vi "Rohwerte skalieren Kalibrieren.vi"(6 "CAL-Daten":T1={"O2 Null"=0.0, "O2 Steil"=[1.0, 1.0, 1.0, 1.0]}, 11 "GasValue":sgl[](array[numeric])) -> (3 "Kalibrierte Rohwerte":sgl[](array[numeric]))   [LabVIEW 2020, in "ABB-EL3000.lvlib" / "PMA.lvlib" / "Kalibrieren.lvlib"]
uses:
  Kalibrieren.lvlib
  Allgemeine VI/CAL-Daten PMA.ctl
  Allgemeine VI/Allgemeine VI.lvlib
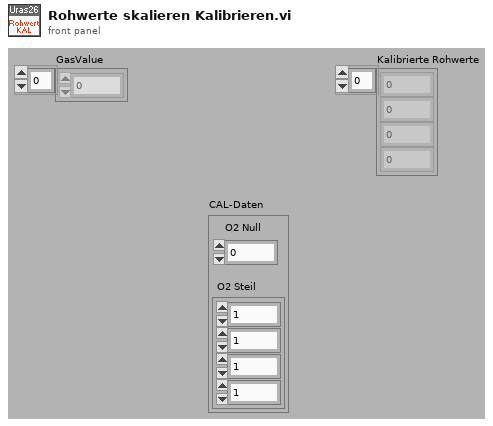
[diagram p1: front panel]
types:
  T1 = typedef "ABB-EL3000.lvlib/Allgemeine VI.lvlib/CAL-Daten PMA.ctl" = cluster{"O2 Null":sgl, "O2 Steil":sgl[]}
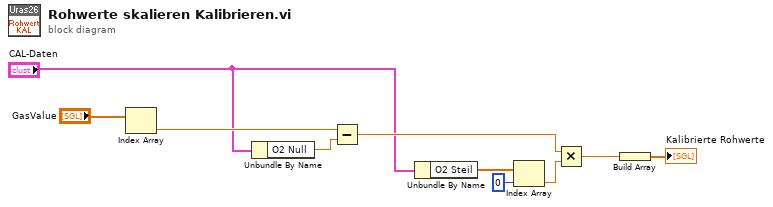
[diagram p0: block diagram]
diagram:
  n1 = Index Array(array="GasValue") -> (element=w3:sgl)  [unwired: 1 in]
  n2 = Unbundle By Name("CAL-Daten") -> ("O2 Null"=w6:sgl)
  n3 = Subtract(x=w3, y=w6) -> (x-y=w7:sgl)
  n4 = Unbundle By Name("CAL-Daten") -> ("O2 Steil"=w8:sgl[])
  n5 = Index Array(array=w8, index=0 ("Index")) -> (element=w9:sgl)
  n6 = Multiply(x=w7, y=w9) -> (x*y=w10:sgl)
  n7 = Build Array(w10) -> (→"Kalibrierte Rohwerte":sgl[])
